vi "LocateSubpanelClasses.vi"(8 "error in (no error)":errorcluster, 9 "Folder Name":string, 10 "Base Path":path, 11 "EmbeddedMainUI in":refnum<class "EmbeddedMainUI.lvclass">) -> (0 "error out":errorcluster, 2 "Class Path":path, 3 "EmbeddedMainUI out":refnum<class "EmbeddedMainUI.lvclass">)   [LabVIEW 2016, in "EmbeddedMainUI.lvclass"]
uses:
  EmbeddedMainUI.lvclass
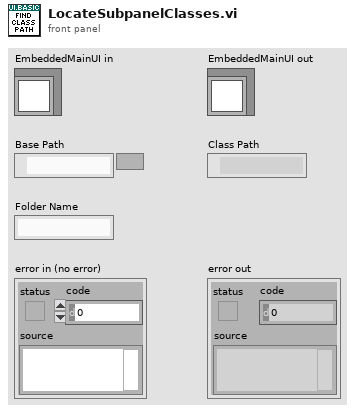
[diagram p1: front panel]
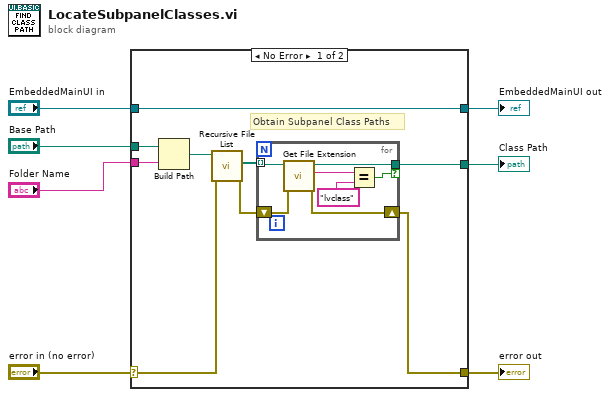
[diagram p0: block diagram]
diagram:
  n1 = case shown="No Error" "error in (no error)" {
    selector: "error in (no error)" -> [w12 w25]
    tunnel: [w11 w25] -> w6
    tunnel: [w16 w24] -> w4
    tunnel: "EmbeddedMainUI in" -> [w16 w24]
    tunnel: [w10 _] -> w3
    tunnel: "Base Path" -> [w9 _]
    tunnel: "Folder Name" -> [w8 _]
    frame No Error {
      # "Obtain Subpanel Class Paths"
      n2 = Build Path(base path=w9, name or relative path=w8) -> (appended path=w15:path)
      n3 = call <vilib>:"Recursive File List.vi"("error in (no error)"=w12, "Folder Path"=w15) -> ("error out"=w13:errorcluster, "All Files in Dir"=w14:path[])  [unwired: 5 in, 3 out]
      n4 = for {
        tunnel: w14 -> [w21] mode=indexing
        tunnel: [w20] -> w10 if=w19
        shift-right: [w17] -> w11
        shift-left: w13 -> [w18]
        n5 = call <vilib>:"Get File Extension.vi"("error in (no error)"=w18, "file"=w21) -> ("error out"=w17:errorcluster, "lowercase file extension"=w23:string, "dup file"=w20:path)  [unwired: 5 in, 2 out]
        n6 = Equal?(x=w23, y="lvclass") -> (x = y?=w19:bool)
      }
    }
    frame Error {
    }
  }
  "error out" <- w6
  "EmbeddedMainUI out" <- w4
  "Class Path" <- w3
